vi "String_StripNullValues.vi"(11 "str in":string) -> (3 "str (stripped)":string)   [LabVIEW 2014, in "hse-misc.lvlib"]
doc: "Removes all NULL values from a string\n\n\n\n____\nHAMPEL SOFTWARE ENGINEERING v0.7.0 (2018-07-16 18:12)"
uses:
  hse-misc.lvlib
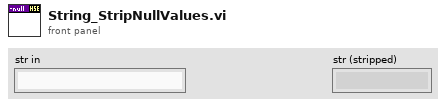
[diagram p1: front panel]
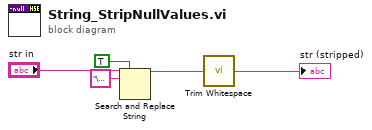
[diagram p0: block diagram]
diagram:
  n1 = Search and Replace String(replace all?=TRUE ("replace all? (F)"), input string="str in", search string="\u0000") -> (result string=w2:string)  [unwired: 5 in, 3 out]
  n2 = call <vilib>:"Trim Whitespace.vi"("string"=w2) -> ("trimmed string"=→"str (stripped)":string)  [unwired: 1 in]
